vi "_Lookup Related Entities.vi"(4 "Relation":T1, 6 "Primary ID":T3, 8 "error in (no error)":errorcluster, 9 "Types":refnum<class "Type.lvclass">[](array[class]), 10 "Entity":refnum<class "Entity.lvclass">, 11 "Database in":refnum<class "Database Platform.lvclass">) -> (0 "error out":errorcluster, 2 "Entities":refnum<class "Entity.lvclass">[](array[class]), 3 "Database out":refnum<class "Database Platform.lvclass">)   [LabVIEW 2020, in "Conditu2.lvlib" / "Database Platform.lvclass"]
uses:
  Database Platform.lvclass
  Columns/Type/Type.lvclass
  Entity/Entity.lvclass
  Entity ID.ctl
  Columns/Relation/Relation Info.ctl
  Relation Mapping.ctl
  Conditu2.lvlib
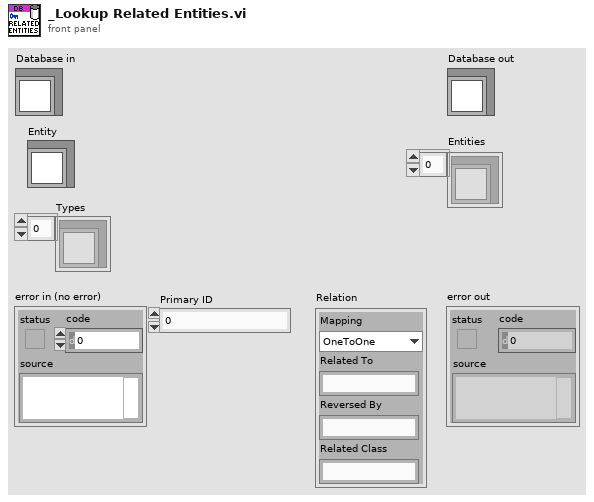
[diagram p1: front panel]
types:
  T1 = typedef "Conditu2.lvlib/Relation Info.ctl" = cluster{"Mapping":T2, "Related To":string, "Reversed By":string, "Related Class":string}
  T2 = typedef "Conditu2.lvlib/Relation Mapping.ctl" = enum16{"OneToOne", "OneToMany", "ManyToOne", "ManyToMany"}
  T3 = typedef "Conditu2.lvlib/Entity ID.ctl" = i64
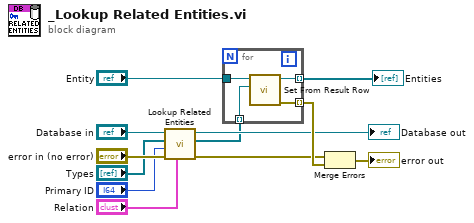
[diagram p0: block diagram]
diagram:
  n1 = call-dynamic "Lookup Related Entities.vi"("Relation"="Relation", "error in (no error)"="error in (no error)", "Primary ID"="Primary ID", "Types"="Types", "Database in"="Database in") -> ("error out"=w9:errorcluster, "Results"=w4:refnum<class "Result Row.lvclass">[], "Database out"=→"Database out":refnum<class "Database Platform.lvclass">)  [unwired: 4 in]
  n2 = for {
    tunnel: w4 -> [w15] mode=indexing
    tunnel: "Entity" -> [w16]
    tunnel: [w14] -> w12 mode=indexing
    tunnel: [w13] -> w2 mode=indexing
    n3 = call "Set From Result Row.vi"("Result Row"=w15, "Entity in"=w16) -> ("error out"=w14:errorcluster, "Entity out"=w13:refnum<class "Entity.lvclass">)  [unwired: 8 in]
  }
  "Entities" <- w2
  n4 = Merge Errors(w9, w12) -> (→"error out":errorcluster)
